vi "Create Event References.vi"(8 "error in (no error)":errorcluster, 11 "Engine in":refnum<class "Engine.lvclass">) -> (0 "error out":errorcluster, 3 "Engine out":refnum<class "Engine.lvclass">)   [LabVIEW 2023, in "Engine.lvlib" / "Engine.lvclass"]
uses:
  Library/Engine.lvclass
  Custom Controls/Faults.ctl
  Custom Controls/Status.ctl
  Custom Controls/AbstractMessage.ctl
  Library/Engine.lvclass/Engine.ctl
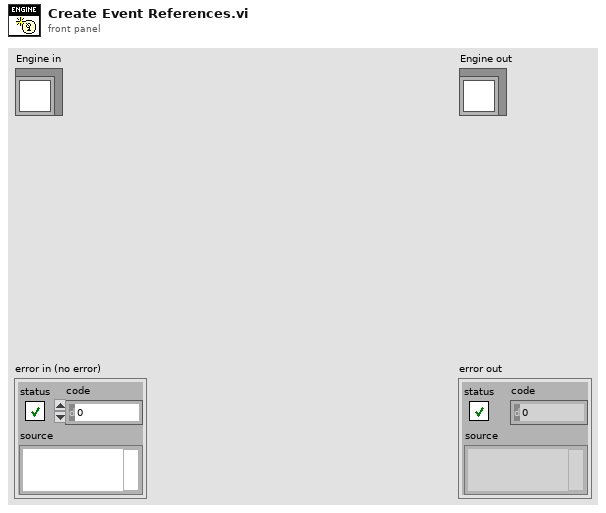
[diagram p1: front panel]
types:
  T1 = typedef "Engine.lvlib/Engine.lvclass/AbstractMessage.ctl" = cluster{"Target":string, "Type":string, "Payload":variant}
  T2 = typedef "Engine.lvlib/Engine.lvclass/Status.ctl" = enum16{"IDLE", "READY", "LAUNCHING", "ERROR", "WARNING", "MANUAL", "AUTOMATION"}
  T3 = typedef "Engine.lvlib/Engine.lvclass/Faults.ctl" = cluster{"Device":string, "Fault":errorcluster}
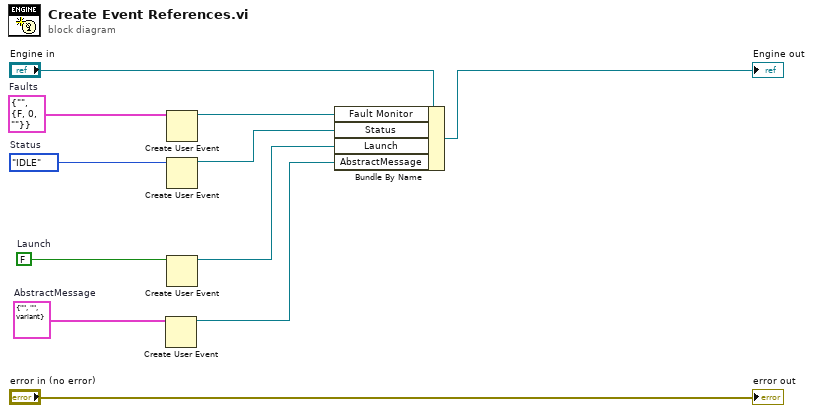
[diagram p0: block diagram]
diagram:
  w3 = T1 {"Target"="", "Type"="", "Payload"=variant}  # AbstractMessage
  w5 = Status."IDLE"  # Status
  w7 = FALSE  # Launch
  w9 = T3 {"Device"="", "Fault"={"status"=FALSE, "code"=0, "source"=""}}  # Faults
  n1 = Create User Event(user event datatype=w3) -> (user event=w1:refnum<user-event>)  [unwired: 1 in, 1 out]
  n2 = Create User Event(user event datatype=w9) -> (user event=w6:refnum<user-event>)  [unwired: 1 in, 1 out]
  n3 = Create User Event(user event datatype=w5) -> (user event=w4:refnum<user-event>)  [unwired: 1 in, 1 out]
  n4 = Create User Event(user event datatype=w7) -> (user event=w2:refnum<user-event>)  [unwired: 1 in, 1 out]
  n5 = Bundle By Name(cluster="Engine in", "Fault Monitor"=w6, "Status"=w4, "Launch"=w2, "AbstractMessage"=w1) -> (→"Engine out":refnum<class "Engine.lvclass">)
  "error out" <- "error in (no error)"
